vi "MU Calibration Is Analog Analyses Valid.vi"(8 "error in (no error)":errorcluster, 11 "AnalyzeResultHandle":T1) -> (0 "error out":errorcluster, 3 "isAnalogAnalysesValid":bool)   [LabVIEW 2017, in "MU_3SL_interface.lvlib"]
uses:
  MU_3SL_interface.lvlib
  handles/CalibrationAnalyzeResultHandle.ctl
  lib/MU_3SL_interface.dll
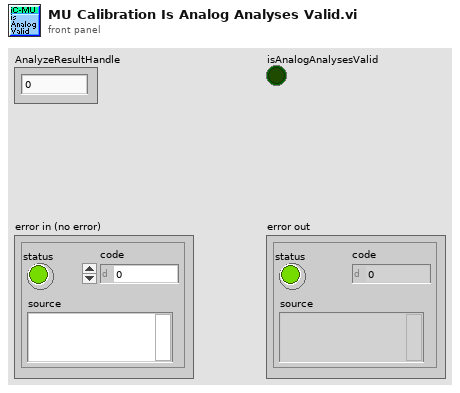
[diagram p1: front panel]
types:
  T1 = typedef "MU_3SL_interface.lvlib/CalibrationAnalyzeResultHandle.ctl" = u64
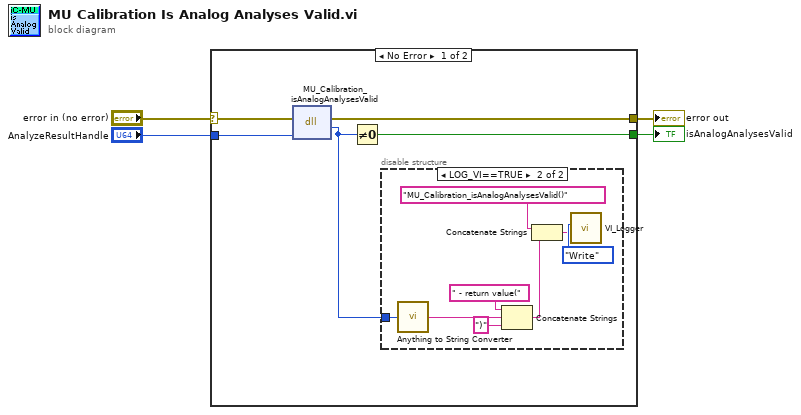
[diagram p0: block diagram]
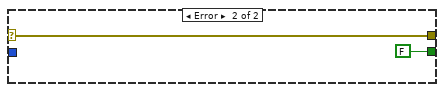
[diagram p3: hidden frame]
diagram:
  n1 = case shown="No Error" "error in (no error)" {
    selector: "error in (no error)" -> [w9 w19]
    tunnel: [w6 FALSE] -> w1
    tunnel: [w7 w19] -> w4
    tunnel: "AnalyzeResultHandle" -> [w8 _]
    frame No Error {
      n2 = dll-call lib="C:/Users/bes/AppData/Roaming/work/mu_9so/icsubmodules/soft_mu_3sl_master/lv_interface/lib/MU_3SL_interface**.*" fn="MU_Calibration_isAnalogAnalysesValid"(error in=w9, "AnalyzeResultHandle"=w8) -> (error out=w7:errorcluster, "isAnalogAnalysesValid"=w5:u8)  [unwired: 3 in, 1 out]
      n3 = Not Equal To 0?(x=w5) -> (x != 0?=w6:bool)
      n4 = disable-structure shown="LOG_VI==TRUE" {
        disable-tunnel: w5 -> [_ w10]
        frame condition #0 {
        }
        frame condition #1 (active) {
          n5 = call "Anything to String Converter.vi"("anything"=w10) -> ("String"=w11:string)
          n6 = Concatenate Strings(" - return value(" ("string"), w11, ")" ("string")) -> (w15:string)
          n7 = Concatenate Strings("MU_Calibration_isAnalogAnalysesValid()" ("Info in"), w15) -> (w14:string)
          n8 = call "VI_Logger.vi"("Action (Read)"=enum16{"Write", "Read"}."Write", "Info in"=w14) -> ()  [unwired: 8 in, 2 out]
        }
      }
    }
    frame Error {
    }
  }
  "error out" <- w4
  "isAnalogAnalysesValid" <- w1
